vi "torres hanoi labview.vi"() -> ()   [LabVIEW 2020]
uses:
  <vilib>/Utility/miscctls.llb/LVPoint32TypeDef.ctl
  <vilib>/Utility/miscctls.llb/LVPositionTypeDef.ctl
  <vilib>/Utility/miscctls.llb/LVBoundsTypeDef.ctl
panel:
  out "Solucion del juego de 5 discos":string
  out "Boolean 3":bool
  out "Solucion del juego de 4 discos":string
  out "Boolean 2":bool
  out "Boolean":bool
  out "solucion del juego 3 discos":string
  out "Position 1":T1
  out "Position 2":T1
  out "Position 3":T1
  out "Position 4":T1
  out "Position 5":T1
  out "Position":T1
  in  "seleccione  numero de discos":u16(ring) items=["3"=3, "4"=4, "5"=5]
  out "Coords":T2
  in  "?":bool
  out "disco5":bool
  out "disco4":bool
  out "disco3":bool
  out "disco2":bool
  out "disco1":bool
  out "Torre 3":bool
  out "Torre 2":bool
  out "Torre 1":bool
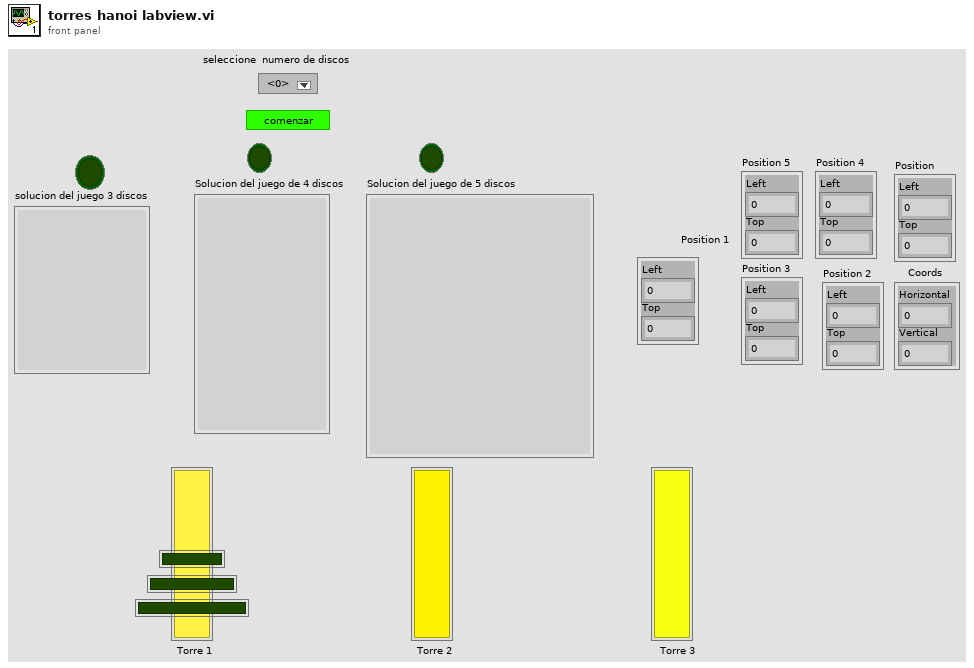
[diagram p1: front panel]
types:
  T1 = typedef "LVPositionTypeDef.ctl" = cluster{"Left":i32, "Top":i32}
  T2 = typedef "LVPoint32TypeDef.ctl" = cluster{"Horizontal":i32, "Vertical":i32}
  T3 = typedef "LVBoundsTypeDef.ctl" = cluster{"Width":u32, "Height":u32}
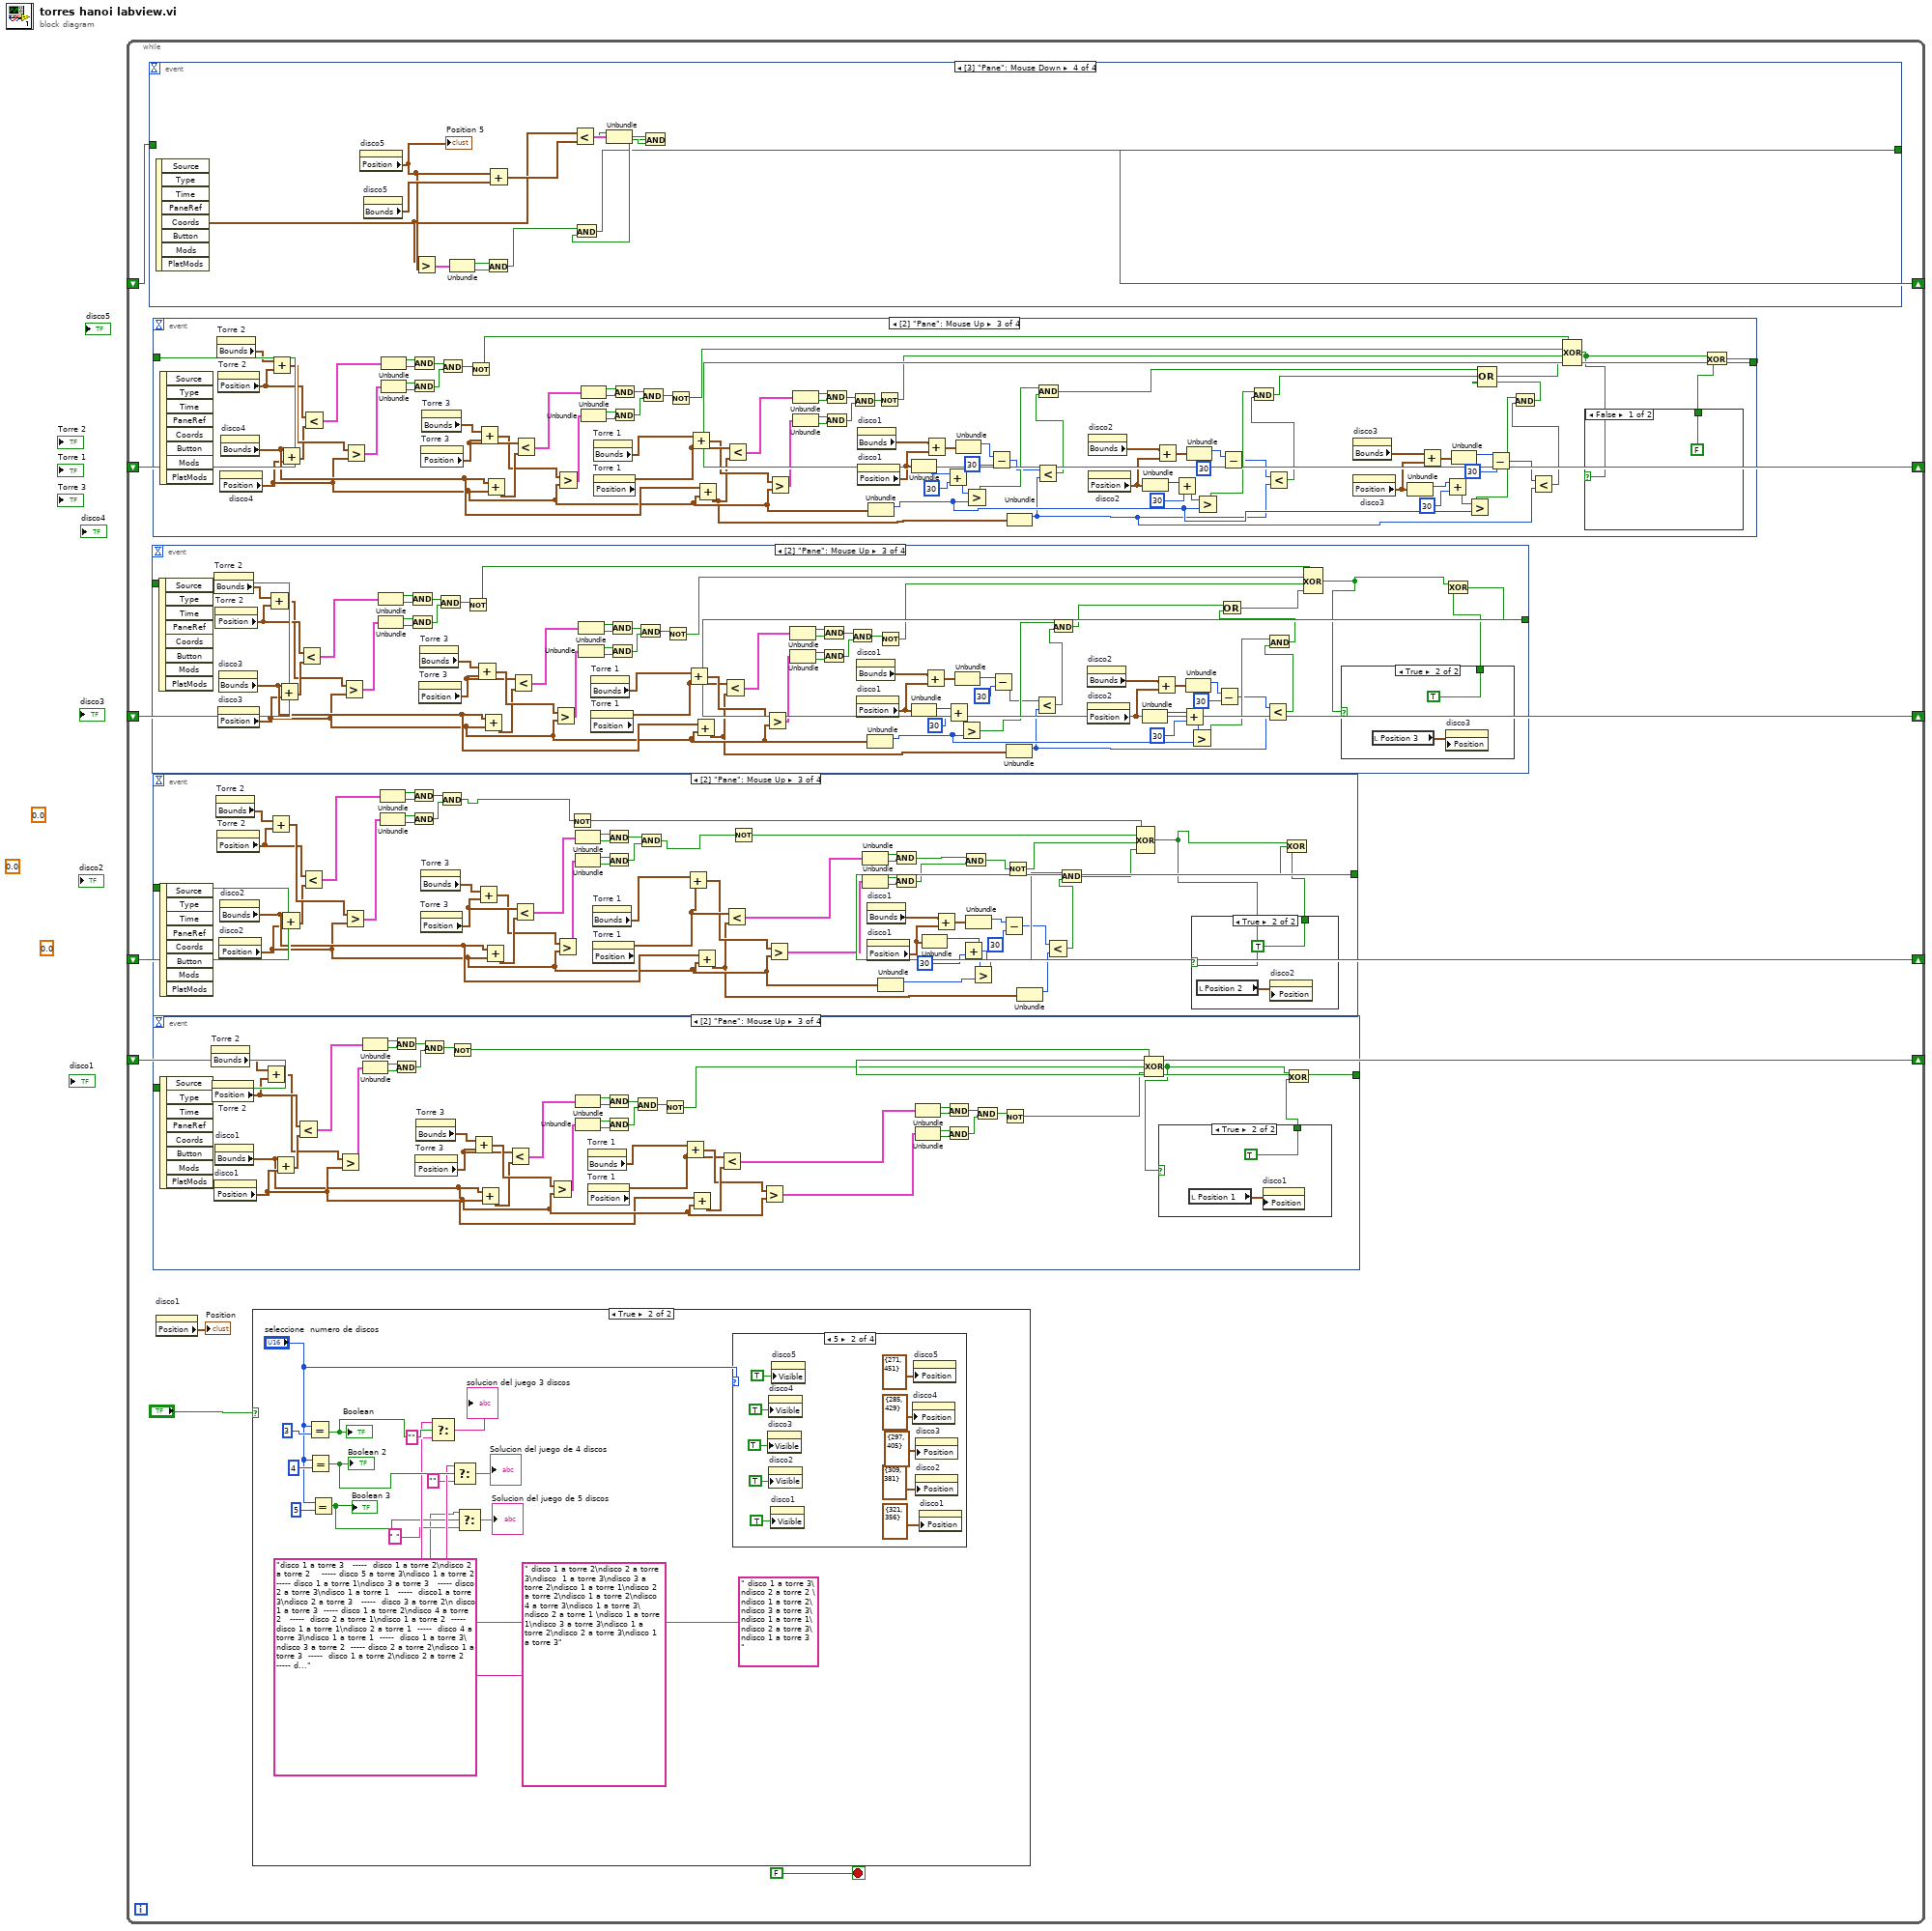
[diagram p0: block diagram]
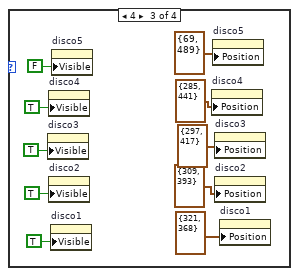
[diagram p4: hidden frame]
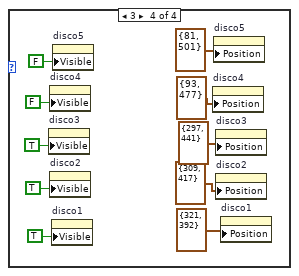
[diagram p5: hidden frame]
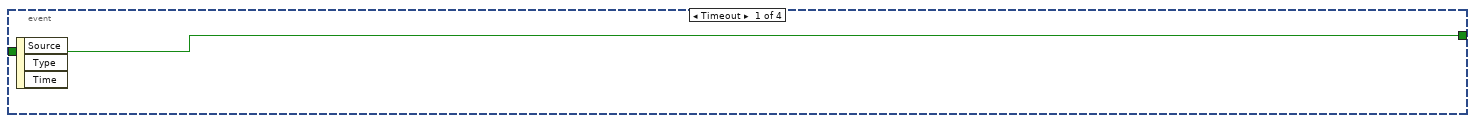
[diagram p6: hidden frame]
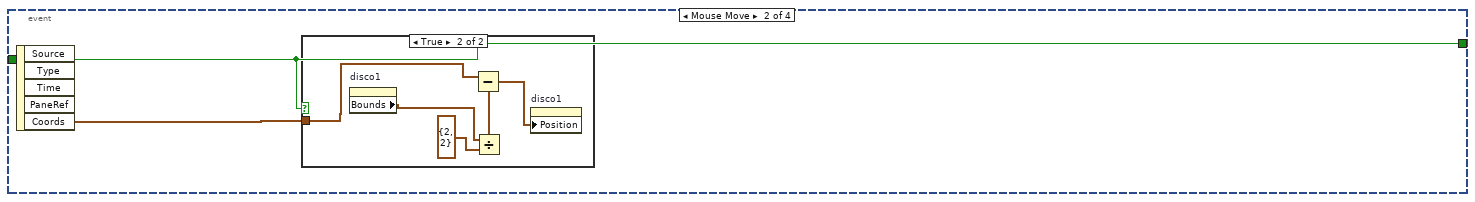
[diagram p7: hidden frame]
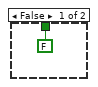
[diagram p9: hidden frame]
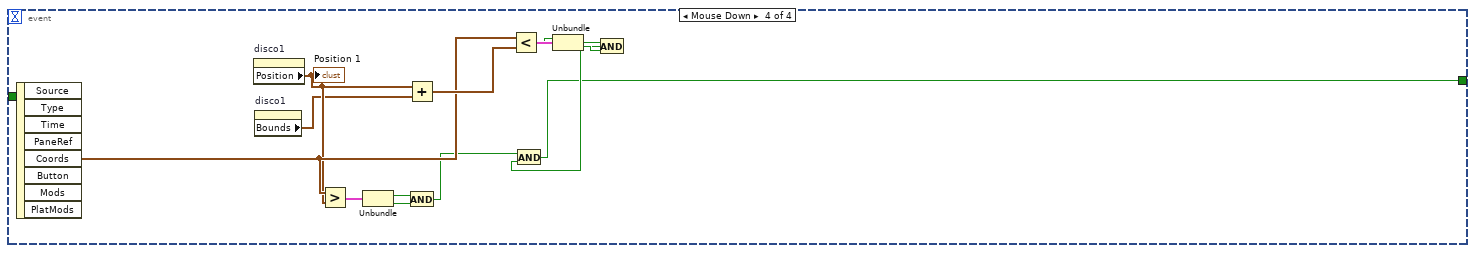
[diagram p10: hidden frame]
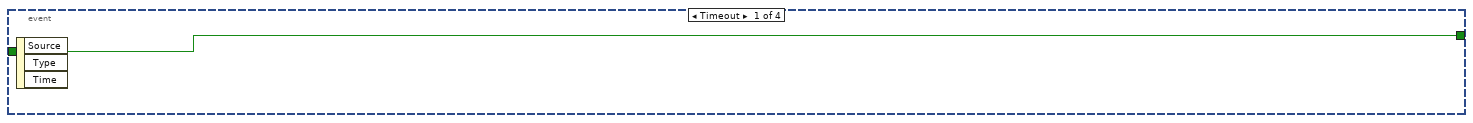
[diagram p11: hidden frame]
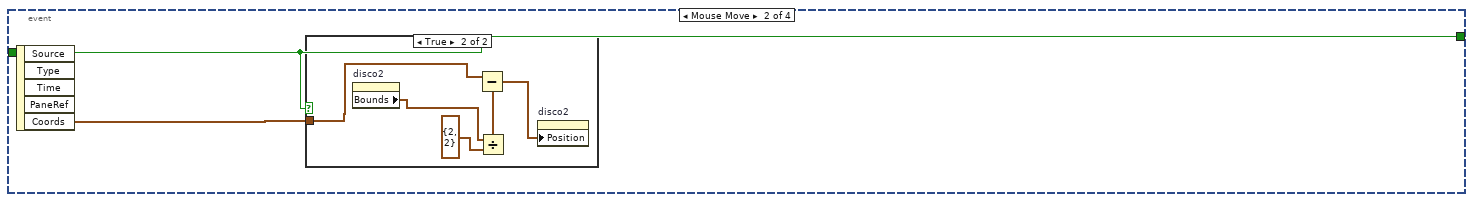
[diagram p12: hidden frame]
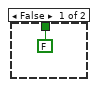
[diagram p14: hidden frame]
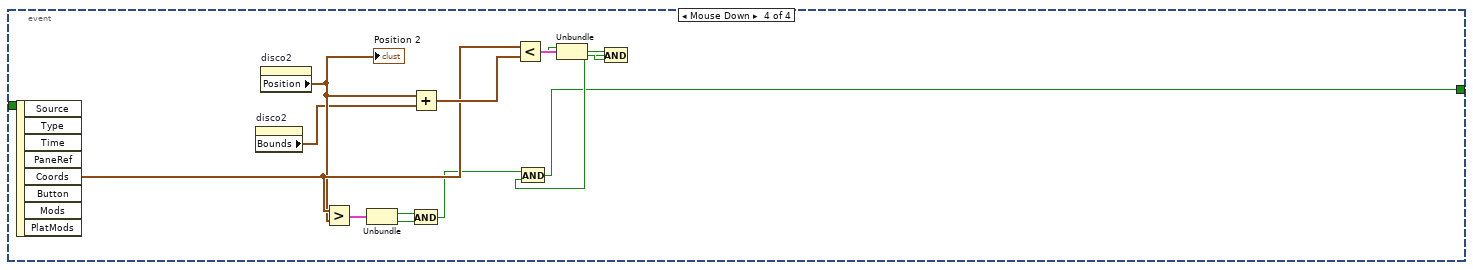
[diagram p15: hidden frame]
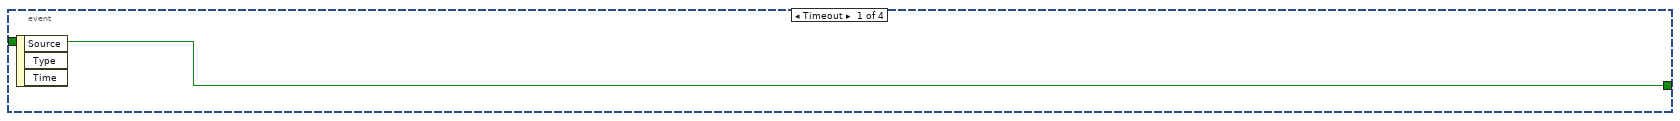
[diagram p16: hidden frame]
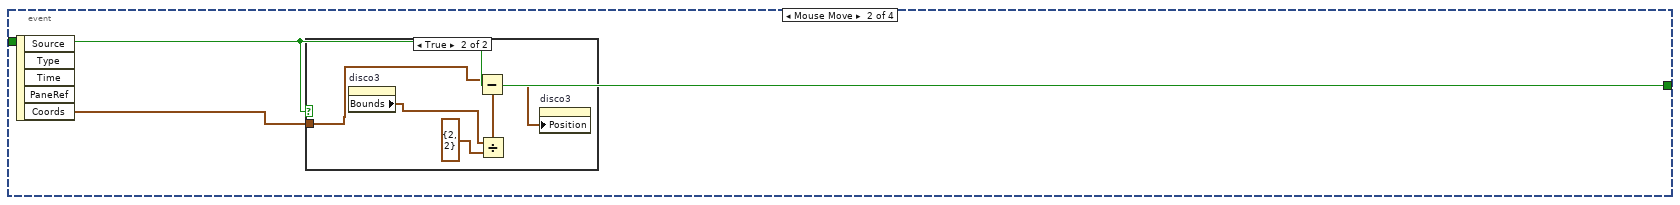
[diagram p17: hidden frame]
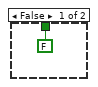
[diagram p19: hidden frame]
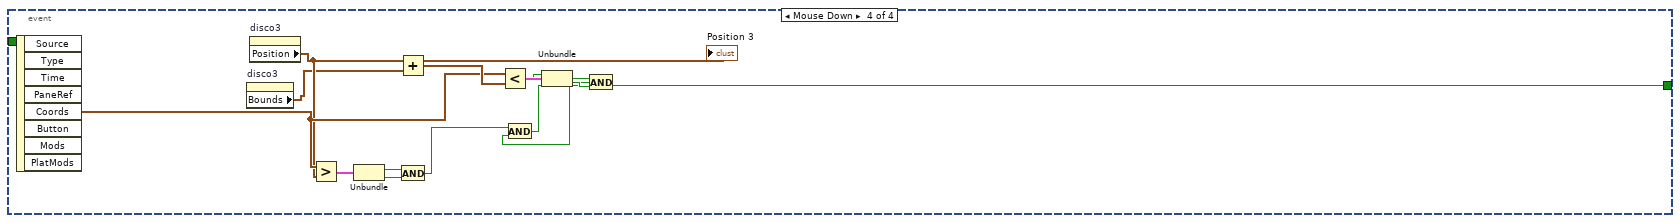
[diagram p20: hidden frame]
diagram:
  (unwired) 0.0 ("final b")
  (unwired) 0.0 ("inicio b")
  (unwired) 0.0 ("medio b")
  n1 = while {
    shift-right: [w11] -> _
    shift-left: _ -> [w12]
    shift-right: [w9] -> _
    shift-left: _ -> [w10]
    shift-right: [w7] -> _
    shift-left: _ -> [w8]
    shift-right: [w5] -> _
    shift-left: _ -> [w6]
    shift-right: [w3] -> _
    shift-left: _ -> [w4]
    stop <- FALSE stop-if-true
    n2 = event shown="[3] \"Pane\": Mouse Down" {
      selector: _ -> [_ _ _ _]
      dyn-events: _ -> [_ _ _ _]
      timeout: _ -> [_ _ _ _]
      tunnel: w12 -> [w424 w425 _ _]
      tunnel: [w424 w425 w485 w533] -> w11
      event Timeout {
        n3 = event-data() -> ()  [unwired: 1 in, 3 out]
      }
      event Mouse Move {
        n4 = event-data() -> ("Coords"=w426:T2)  [unwired: 1 in, 4 out]
        n5 = case shown="True" w425 {
          tunnel: w426 -> [_ w429]
          frame False {
          }
          frame True {
            n6 = property on="disco5" class="Bool (strict)"() -> ("Bounds"=w431:T3)  [unwired: 2 in, 2 out]
            n7 = Divide(x=w431, y=T3 {"Width"=2, "Height"=2}) -> (x/y=w428:cluster{"Width":dbl, "Height":dbl})
            n8 = Subtract(x=w429, y=w428) -> (x-y=w427:cluster{dbl, dbl})
            n9 = property on="disco5" class="Bool (strict)"("Position"=w427) -> ()  [unwired: 2 in, 2 out]
            "Coords" <- w429
          }
        }
      }
      event Mouse Up {
        n10 = event-data() -> ()  [unwired: 1 in, 8 out]
        n11 = property on="Torre 2" class="Bool (strict)"() -> ("Bounds"=w520:T3)  [unwired: 2 in, 2 out]
        n12 = property on="Torre 2" class="Bool (strict)"() -> ("Position"=w519:T1)  [unwired: 2 in, 2 out]
        n13 = property on="disco5" class="Bool (strict)"() -> ("Position"=w473:T1)  [unwired: 2 in, 2 out]
        n14 = property on="disco5" class="Bool (strict)"() -> ("Bounds"=w491:T3)  [unwired: 2 in, 2 out]
        n15 = Add(x=w520, y=w519) -> (x+y=w518:T3)
        n16 = Add(x=w491, y=w473) -> (x+y=w523:T3)
        n17 = Less?(x=w519, y=w523) -> (x < y?=w522:cluster{bool, bool})
        n18 = Greater?(x=w518, y=w473) -> (0:w521:cluster{bool, bool})
        n19 = Unbundle(w522) -> (w527:bool, w526:bool)
        n20 = Unbundle(w521) -> (w529:bool, w528:bool)
        n21 = And(x=w527, y=w526) -> (x .and. y?=w524:bool)
        n22 = And(x=w529, y=w528) -> (x .and. y?=w525:bool)
        n23 = property on="Torre 3" class="Bool (strict)"() -> ("Position"=w504:T1)  [unwired: 2 in, 2 out]
        n24 = property on="Torre 3" class="Bool (strict)"() -> ("Bounds"=w505:T3)  [unwired: 2 in, 2 out]
        n25 = And(x=w524, y=w525) -> (x .and. y?=w517:bool)
        n26 = Not(x=w517) -> (.not. x?=w488:bool)
        n27 = Add(x=w505, y=w504) -> (x+y=w515:T3)
        n28 = Add(x=w491, y=w473) -> (x+y=w512:T3)
        n29 = Less?(x=w504, y=w512) -> (x < y?=w513:cluster{bool, bool})
        n30 = Greater?(x=w515, y=w473) -> (0:w514:cluster{bool, bool})
        n31 = Unbundle(w513) -> (w508:bool, w509:bool)
        n32 = Unbundle(w514) -> (w506:bool, w507:bool)
        n33 = property on="Torre 1" class="Bool (strict)"() -> ("Bounds"=w493:T3)  [unwired: 2 in, 2 out]
        n34 = property on="Torre 1" class="Bool (strict)"() -> ("Position"=w492:T1)  [unwired: 2 in, 2 out]
        n35 = And(x=w508, y=w509) -> (x .and. y?=w511:bool)
        n36 = And(x=w506, y=w507) -> (x .and. y?=w510:bool)
        n37 = And(x=w511, y=w510) -> (x .and. y?=w516:bool)
        n38 = Not(x=w516) -> (.not. x?=w489:bool)
        n39 = Add(x=w493, y=w492) -> (x+y=w495:T3)
        n40 = Add(x=w491, y=w473) -> (x+y=w472:T3)
        n41 = Less?(x=w492, y=w472) -> (x < y?=w497:cluster{bool, bool})
        n42 = Greater?(x=w495, y=w473) -> (0:w496:cluster{bool, bool})
        n43 = Unbundle(w497) -> (w501:bool, w500:bool)
        n44 = Unbundle(w496) -> (w503:bool, w502:bool)
        n45 = property on="disco1" class="Bool (strict)"() -> ("Bounds"=w479:T3)  [unwired: 2 in, 2 out]
        n46 = property on="disco1" class="Bool (strict)"() -> ("Position"=w480:T1)  [unwired: 2 in, 2 out]
        n47 = Unbundle(w473) -> ("Left"=w462:i32)  [unwired: 1 out]
        n48 = And(x=w501, y=w500) -> (x .and. y?=w498:bool)
        n49 = And(x=w503, y=w502) -> (x .and. y?=w499:bool)
        n50 = And(x=w498, y=w499) -> (x .and. y?=w494:bool)
        n51 = Unbundle(w480) -> ("Left"=w460:i32)  [unwired: 1 out]
        n52 = Add(x=w479, y=w480) -> (x+y=w481:T3)
        n53 = Not(x=w494) -> (.not. x?=w490:bool)
        n54 = Add(x=w460, y=30) -> (x+y=w458:i32)
        n55 = Greater?(x=w458, y=w462) -> (0:w475:bool)
        n56 = Unbundle(w481) -> ("Width"=w457:u32)  [unwired: 1 out]
        n57 = Subtract(x=w457, y=u32 30) -> (x-y=w455:u32)
        n58 = Unbundle(w472) -> ("Width"=w461:u32)  [unwired: 1 out]
        n59 = Less?(x=w455, y=w461) -> (x < y?=w474:bool)
        n60 = And(x=w475, y=w474) -> (x .and. y?=w432:bool)
        n61 = property on="disco2" class="Bool (strict)"() -> ("Bounds"=w478:T3)  [unwired: 2 in, 2 out]
        n62 = property on="disco2" class="Bool (strict)"() -> ("Position"=w477:T1)  [unwired: 2 in, 2 out]
        n63 = Unbundle(w477) -> ("Left"=w453:i32)  [unwired: 1 out]
        n64 = Add(x=w478, y=w477) -> (x+y=w476:T3)
        n65 = Add(x=w453, y=30) -> (x+y=w454:i32)
        n66 = Unbundle(w476) -> ("Width"=w451:u32)  [unwired: 1 out]
        n67 = Greater?(x=w454, y=w462) -> (0:w471:bool)
        n68 = Subtract(x=w451, y=u32 30) -> (x-y=w450:u32)
        n69 = Less?(x=w450, y=w461) -> (x < y?=w470:bool)
        n70 = And(x=w471, y=w470) -> (x .and. y?=w433:bool)
        n71 = property on="disco3" class="Bool (strict)"() -> ("Bounds"=w482:T3)  [unwired: 2 in, 2 out]
        n72 = property on="disco3" class="Bool (strict)"() -> ("Position"=w483:T1)  [unwired: 2 in, 2 out]
        n73 = Unbundle(w483) -> ("Left"=w448:i32)  [unwired: 1 out]
        n74 = Add(x=w482, y=w483) -> (x+y=w484:T3)
        n75 = Add(x=w448, y=30) -> (x+y=w447:i32)
        n76 = Unbundle(w484) -> ("Width"=w445:u32)  [unwired: 1 out]
        n77 = Greater?(x=w447, y=w462) -> (0:w469:bool)
        n78 = Subtract(x=w445, y=u32 30) -> (x-y=w444:u32)
        n79 = Less?(x=w444, y=w461) -> (x < y?=w468:bool)
        n80 = And(x=w469, y=w468) -> (x .and. y?=w434:bool)
        n81 = property on="disco4" class="Bool (strict)"() -> ("Bounds"=w465:T3)  [unwired: 2 in, 2 out]
        n82 = property on="disco4" class="Bool (strict)"() -> ("Position"=w464:T1)  [unwired: 2 in, 2 out]
        n83 = Unbundle(w464) -> ("Left"=w442:i32)  [unwired: 1 out]
        n84 = Add(x=w465, y=w464) -> (x+y=w463:T3)
        n85 = Add(x=w442, y=30) -> (x+y=w441:i32)
        n86 = Greater?(x=w441, y=w462) -> (0:w466:bool)
        n87 = Unbundle(w463) -> ("Width"=w439:u32)  [unwired: 1 out]
        n88 = Subtract(x=w439, y=u32 30) -> (x-y=w437:u32)
        n89 = Less?(x=w437, y=w461) -> (x < y?=w467:bool)
        n90 = And(x=w466, y=w467) -> (x .and. y?=w435:bool)
        n91 = Compound Arithmetic op=OR(w432, w433, w434, w435) -> (w436:bool)
        n92 = Compound Arithmetic op=XOR(w488, w489, w490, w436) -> (w486:bool)
        n93 = case shown="True" w486 {
          tunnel: [FALSE ("Accepted?") TRUE ("Accepted?")] -> w487
          frame False {
          }
          frame True {
            n94 = local read "Position 5"() -> (w532:T1)
            n95 = property on="disco5" class="Bool (strict)"("Position"=w532) -> ()  [unwired: 2 in, 2 out]
          }
        }
        n96 = Exclusive Or(1:w487, 2:w486) -> (0:w485:bool)
      }
      event Mouse Down {
        n97 = event-data() -> ("Coords"=w542:T2)  [unwired: 1 in, 7 out]
        n98 = property on="disco5" class="Bool (strict)"() -> ("Position"=w544:T1)  [unwired: 2 in, 2 out]
        "Position 5" <- w544
        n99 = property on="disco5" class="Bool (strict)"() -> ("Bounds"=w545:T3)  [unwired: 2 in, 2 out]
        n100 = Greater?(x=w542, y=w544) -> (0:w541:cluster{bool, bool})
        n101 = Unbundle(w541) -> (w537:bool, w536:bool)
        n102 = Add(x=w544, y=w545) -> (x+y=w543:T3)
        n103 = And(x=w537, y=w536) -> (x .and. y?=w534:bool)
        n104 = Less?(x=w542, y=w543) -> (x < y?=w540:cluster{bool, bool})
        n105 = Unbundle(w540) -> (w539:bool, w538:bool)
        n106 = And(x=w539, y=w538) -> (x .and. y?=w535:bool)
        n107 = And(x=w534, y=w535) -> (x .and. y?=w533:bool)
      }
    }
    n108 = event shown="[2] \"Pane\": Mouse Up" {
      selector: _ -> [_ _ _ _]
      dyn-events: _ -> [_ _ _ _]
      timeout: _ -> [_ _ _ _]
      tunnel: w8 -> [w216 w217 _ _]
      tunnel: [w216 w217 w253 w303] -> w7
      event Timeout {
        n109 = event-data() -> ()  [unwired: 1 in, 3 out]
      }
      event Mouse Move {
        n110 = event-data() -> ("Coords"=w218:T2)  [unwired: 1 in, 4 out]
        n111 = case shown="True" w217 {
          tunnel: w218 -> [_ w222]
          frame False {
          }
          frame True {
            n112 = property on="disco3" class="Bool (strict)"() -> ("Bounds"=w220:T3)  [unwired: 2 in, 2 out]
            n113 = Divide(x=w220, y=T3 {"Width"=2, "Height"=2}) -> (x/y=w221:cluster{"Width":dbl, "Height":dbl})
            n114 = Subtract(x=w222, y=w221) -> (x-y=w219:cluster{dbl, dbl})
            n115 = property on="disco3" class="Bool (strict)"("Position"=w219) -> ()  [unwired: 2 in, 2 out]
          }
        }
      }
      event Mouse Up {
        n116 = event-data() -> ()  [unwired: 1 in, 8 out]
        n117 = property on="Torre 2" class="Bool (strict)"() -> ("Bounds"=w288:T3)  [unwired: 2 in, 2 out]
        n118 = property on="Torre 2" class="Bool (strict)"() -> ("Position"=w287:T1)  [unwired: 2 in, 2 out]
        n119 = property on="disco3" class="Bool (strict)"() -> ("Position"=w249:T1)  [unwired: 2 in, 2 out]
        n120 = property on="disco3" class="Bool (strict)"() -> ("Bounds"=w259:T3)  [unwired: 2 in, 2 out]
        n121 = Add(x=w288, y=w287) -> (x+y=w286:T3)
        n122 = Add(x=w259, y=w249) -> (x+y=w291:T3)
        n123 = Less?(x=w287, y=w291) -> (x < y?=w290:cluster{bool, bool})
        n124 = Greater?(x=w286, y=w249) -> (0:w289:cluster{bool, bool})
        n125 = Unbundle(w290) -> (w295:bool, w294:bool)
        n126 = Unbundle(w289) -> (w297:bool, w296:bool)
        n127 = And(x=w295, y=w294) -> (x .and. y?=w292:bool)
        n128 = And(x=w297, y=w296) -> (x .and. y?=w293:bool)
        n129 = property on="Torre 3" class="Bool (strict)"() -> ("Position"=w272:T1)  [unwired: 2 in, 2 out]
        n130 = property on="Torre 3" class="Bool (strict)"() -> ("Bounds"=w273:T3)  [unwired: 2 in, 2 out]
        n131 = And(x=w292, y=w293) -> (x .and. y?=w285:bool)
        n132 = Not(x=w285) -> (.not. x?=w256:bool)
        n133 = Add(x=w273, y=w272) -> (x+y=w283:T3)
        n134 = Add(x=w259, y=w249) -> (x+y=w280:T3)
        n135 = Less?(x=w272, y=w280) -> (x < y?=w281:cluster{bool, bool})
        n136 = Greater?(x=w283, y=w249) -> (0:w282:cluster{bool, bool})
        n137 = Unbundle(w281) -> (w276:bool, w277:bool)
        n138 = Unbundle(w282) -> (w274:bool, w275:bool)
        n139 = property on="Torre 1" class="Bool (strict)"() -> ("Bounds"=w261:T3)  [unwired: 2 in, 2 out]
        n140 = property on="Torre 1" class="Bool (strict)"() -> ("Position"=w260:T1)  [unwired: 2 in, 2 out]
        n141 = And(x=w276, y=w277) -> (x .and. y?=w279:bool)
        n142 = And(x=w274, y=w275) -> (x .and. y?=w278:bool)
        n143 = And(x=w279, y=w278) -> (x .and. y?=w284:bool)
        n144 = Not(x=w284) -> (.not. x?=w257:bool)
        n145 = Add(x=w261, y=w260) -> (x+y=w263:T3)
        n146 = Add(x=w259, y=w249) -> (x+y=w248:T3)
        n147 = Less?(x=w260, y=w248) -> (x < y?=w265:cluster{bool, bool})
        n148 = Greater?(x=w263, y=w249) -> (0:w264:cluster{bool, bool})
        n149 = Unbundle(w265) -> (w269:bool, w268:bool)
        n150 = Unbundle(w264) -> (w271:bool, w270:bool)
        n151 = And(x=w269, y=w268) -> (x .and. y?=w266:bool)
        n152 = And(x=w271, y=w270) -> (x .and. y?=w267:bool)
        n153 = And(x=w266, y=w267) -> (x .and. y?=w262:bool)
        n154 = property on="disco1" class="Bool (strict)"() -> ("Bounds"=w250:T3)  [unwired: 2 in, 2 out]
        n155 = property on="disco1" class="Bool (strict)"() -> ("Position"=w251:T1)  [unwired: 2 in, 2 out]
        n156 = Unbundle(w249) -> ("Left"=w242:i32)  [unwired: 1 out]
        n157 = Not(x=w262) -> (.not. x?=w258:bool)
        n158 = Unbundle(w251) -> ("Left"=w238:i32)  [unwired: 1 out]
        n159 = Add(x=w250, y=w251) -> (x+y=w252:T3)
        n160 = Add(x=w238, y=30) -> (x+y=w237:i32)
        n161 = Unbundle(w252) -> ("Width"=w234:u32)  [unwired: 1 out]
        n162 = Greater?(x=w237, y=w242) -> (0:w247:bool)
        n163 = Subtract(x=w234, y=u32 30) -> (x-y=w235:u32)
        n164 = Unbundle(w248) -> ("Width"=w241:u32)  [unwired: 1 out]
        n165 = Less?(x=w235, y=w241) -> (x < y?=w246:bool)
        n166 = And(x=w247, y=w246) -> (x .and. y?=w225:bool)
        n167 = property on="disco2" class="Bool (strict)"() -> ("Bounds"=w245:T3)  [unwired: 2 in, 2 out]
        n168 = property on="disco2" class="Bool (strict)"() -> ("Position"=w244:T1)  [unwired: 2 in, 2 out]
        n169 = Unbundle(w244) -> ("Left"=w232:i32)  [unwired: 1 out]
        n170 = Add(x=w245, y=w244) -> (x+y=w243:T3)
        n171 = Add(x=w232, y=30) -> (x+y=w231:i32)
        n172 = Unbundle(w243) -> ("Width"=w229:u32)  [unwired: 1 out]
        n173 = Greater?(x=w231, y=w242) -> (0:w239:bool)
        n174 = Subtract(x=w229, y=u32 30) -> (x-y=w228:u32)
        n175 = Less?(x=w228, y=w241) -> (x < y?=w240:bool)
        n176 = And(x=w239, y=w240) -> (x .and. y?=w226:bool)
        n177 = Or(x=w225, y=w226) -> (x .or. y?=w224:bool)
        n178 = Compound Arithmetic op=XOR(w256, w257, w258, w224) -> (w254:bool)
        n179 = case shown="True" w254 {
          tunnel: [FALSE ("Accepted?") TRUE ("Accepted?")] -> w255
          frame False {
          }
          frame True {
            n180 = local read "Position 3"() -> (w300:T1)
            n181 = property on="disco3" class="Bool (strict)"("Position"=w300) -> ()  [unwired: 2 in, 2 out]
          }
        }
        n182 = Exclusive Or(1:w255, 2:w254) -> (0:w253:bool)
      }
      event Mouse Down {
        n183 = event-data() -> ("Coords"=w312:T2)  [unwired: 1 in, 7 out]
        n184 = property on="disco3" class="Bool (strict)"() -> ("Bounds"=w301:T3)  [unwired: 2 in, 2 out]
        n185 = property on="disco3" class="Bool (strict)"() -> ("Position"=w302:T1)  [unwired: 2 in, 2 out]
        "Position 3" <- w302
        n186 = Greater?(x=w312, y=w302) -> (0:w311:cluster{bool, bool})
        n187 = Unbundle(w311) -> (w307:bool, w306:bool)
        n188 = Add(x=w302, y=w301) -> (x+y=w313:T3)
        n189 = And(x=w307, y=w306) -> (x .and. y?=w304:bool)
        n190 = Less?(x=w312, y=w313) -> (x < y?=w310:cluster{bool, bool})
        n191 = Unbundle(w310) -> (w309:bool, w308:bool)
        n192 = And(x=w309, y=w308) -> (x .and. y?=w305:bool)
        n193 = And(x=w304, y=w305) -> (x .and. y?=w303:bool)
      }
    }
    n194 = event shown="[2] \"Pane\": Mouse Up" {
      selector: _ -> [_ _ _ _]
      dyn-events: _ -> [_ _ _ _]
      timeout: _ -> [_ _ _ _]
      tunnel: w10 -> [w314 w315 _ _]
      tunnel: [w314 w315 w364 w413] -> w9
      event Timeout {
        n195 = event-data() -> ()  [unwired: 1 in, 3 out]
      }
      event Mouse Move {
        n196 = event-data() -> ("Coords"=w316:T2)  [unwired: 1 in, 4 out]
        n197 = case shown="True" w315 {
          tunnel: w316 -> [_ w317]
          frame False {
          }
          frame True {
            n198 = property on="disco4" class="Bool (strict)"() -> ("Bounds"=w319:T3)  [unwired: 2 in, 2 out]
            n199 = Divide(x=w319, y=T3 {"Width"=2, "Height"=2}) -> (x/y=w320:cluster{"Width":dbl, "Height":dbl})
            n200 = Subtract(x=w317, y=w320) -> (x-y=w318:cluster{dbl, dbl})
            n201 = property on="disco4" class="Bool (strict)"("Position"=w318) -> ()  [unwired: 2 in, 2 out]
          }
        }
      }
      event Mouse Up {
        n202 = event-data() -> ()  [unwired: 1 in, 8 out]
        n203 = property on="Torre 2" class="Bool (strict)"() -> ("Bounds"=w374:T3)  [unwired: 2 in, 2 out]
        n204 = property on="Torre 2" class="Bool (strict)"() -> ("Position"=w375:T1)  [unwired: 2 in, 2 out]
        n205 = property on="disco4" class="Bool (strict)"() -> ("Position"=w353:T1)  [unwired: 2 in, 2 out]
        n206 = property on="disco4" class="Bool (strict)"() -> ("Bounds"=w403:T3)  [unwired: 2 in, 2 out]
        n207 = Add(x=w374, y=w375) -> (x+y=w376:T3)
        n208 = Add(x=w403, y=w353) -> (x+y=w371:T3)
        n209 = Less?(x=w375, y=w371) -> (x < y?=w372:cluster{bool, bool})
        n210 = Greater?(x=w376, y=w353) -> (0:w373:cluster{bool, bool})
        n211 = Unbundle(w372) -> (w367:bool, w368:bool)
        n212 = Unbundle(w373) -> (w365:bool, w366:bool)
        n213 = And(x=w367, y=w368) -> (x .and. y?=w370:bool)
        n214 = And(x=w365, y=w366) -> (x .and. y?=w369:bool)
        n215 = property on="Torre 3" class="Bool (strict)"() -> ("Position"=w390:T1)  [unwired: 2 in, 2 out]
        n216 = property on="Torre 3" class="Bool (strict)"() -> ("Bounds"=w389:T3)  [unwired: 2 in, 2 out]
        n217 = And(x=w370, y=w369) -> (x .and. y?=w377:bool)
        n218 = Not(x=w377) -> (.not. x?=w405:bool)
        n219 = Add(x=w389, y=w390) -> (x+y=w379:T3)
        n220 = Add(x=w403, y=w353) -> (x+y=w382:T3)
        n221 = Less?(x=w390, y=w382) -> (x < y?=w381:cluster{bool, bool})
        n222 = Greater?(x=w379, y=w353) -> (0:w380:cluster{bool, bool})
        n223 = Unbundle(w381) -> (w386:bool, w385:bool)
        n224 = Unbundle(w380) -> (w388:bool, w387:bool)
        n225 = property on="Torre 1" class="Bool (strict)"() -> ("Bounds"=w401:T3)  [unwired: 2 in, 2 out]
        n226 = property on="Torre 1" class="Bool (strict)"() -> ("Position"=w402:T1)  [unwired: 2 in, 2 out]
        n227 = And(x=w386, y=w385) -> (x .and. y?=w383:bool)
        n228 = And(x=w388, y=w387) -> (x .and. y?=w384:bool)
        n229 = And(x=w383, y=w384) -> (x .and. y?=w378:bool)
        n230 = Not(x=w378) -> (.not. x?=w404:bool)
        n231 = Add(x=w401, y=w402) -> (x+y=w399:T3)
        n232 = Add(x=w403, y=w353) -> (x+y=w352:T3)
        n233 = Less?(x=w402, y=w352) -> (x < y?=w397:cluster{bool, bool})
        n234 = Greater?(x=w399, y=w353) -> (0:w398:cluster{bool, bool})
        n235 = Unbundle(w397) -> (w393:bool, w394:bool)
        n236 = Unbundle(w398) -> (w391:bool, w392:bool)
        n237 = And(x=w393, y=w394) -> (x .and. y?=w396:bool)
        n238 = And(x=w391, y=w392) -> (x .and. y?=w395:bool)
        n239 = And(x=w396, y=w395) -> (x .and. y?=w400:bool)
        n240 = property on="disco1" class="Bool (strict)"() -> ("Bounds"=w360:T3)  [unwired: 2 in, 2 out]
        n241 = property on="disco1" class="Bool (strict)"() -> ("Position"=w359:T1)  [unwired: 2 in, 2 out]
        n242 = Unbundle(w353) -> ("Left"=w348:i32)  [unwired: 1 out]
        n243 = Not(x=w400) -> (.not. x?=w323:bool)
        n244 = Unbundle(w359) -> ("Left"=w344:i32)  [unwired: 1 out]
        n245 = Add(x=w360, y=w359) -> (x+y=w358:T3)
        n246 = Add(x=w344, y=30) -> (x+y=w342:i32)
        n247 = Unbundle(w358) -> ("Width"=w341:u32)  [unwired: 1 out]
        n248 = Greater?(x=w342, y=w348) -> (0:w355:bool)
        n249 = Subtract(x=w341, y=u32 30) -> (x-y=w340:u32)
        n250 = Unbundle(w352) -> ("Width"=w347:u32)  [unwired: 1 out]
        n251 = Less?(x=w340, y=w347) -> (x < y?=w354:bool)
        n252 = And(x=w355, y=w354) -> (x .and. y?=w324:bool)
        n253 = property on="disco2" class="Bool (strict)"() -> ("Bounds"=w361:T3)  [unwired: 2 in, 2 out]
        n254 = property on="disco2" class="Bool (strict)"() -> ("Position"=w362:T1)  [unwired: 2 in, 2 out]
        n255 = Unbundle(w362) -> ("Left"=w337:i32)  [unwired: 1 out]
        n256 = Add(x=w361, y=w362) -> (x+y=w363:T3)
        n257 = Add(x=w337, y=30) -> (x+y=w338:i32)
        n258 = Unbundle(w363) -> ("Width"=w335:u32)  [unwired: 1 out]
        n259 = Greater?(x=w338, y=w348) -> (0:w357:bool)
        n260 = Subtract(x=w335, y=u32 30) -> (x-y=w333:u32)
        n261 = Less?(x=w333, y=w347) -> (x < y?=w356:bool)
        n262 = And(x=w357, y=w356) -> (x .and. y?=w325:bool)
        n263 = property on="disco3" class="Bool (strict)"() -> ("Bounds"=w351:T3)  [unwired: 2 in, 2 out]
        n264 = property on="disco3" class="Bool (strict)"() -> ("Position"=w350:T1)  [unwired: 2 in, 2 out]
        n265 = Unbundle(w350) -> ("Left"=w332:i32)  [unwired: 1 out]
        n266 = Add(x=w351, y=w350) -> (x+y=w349:T3)
        n267 = Add(x=w332, y=30) -> (x+y=w331:i32)
        n268 = Unbundle(w349) -> ("Width"=w329:u32)  [unwired: 1 out]
        n269 = Greater?(x=w331, y=w348) -> (0:w346:bool)
        n270 = Subtract(x=w329, y=u32 30) -> (x-y=w328:u32)
        n271 = Less?(x=w328, y=w347) -> (x < y?=w345:bool)
        n272 = And(x=w346, y=w345) -> (x .and. y?=w326:bool)
        n273 = Compound Arithmetic op=OR(w324, w325, w326) -> (w322:bool)
        n274 = Compound Arithmetic op=XOR(w405, w404, w323, w322) -> (w407:bool)
        n275 = case shown="False" w407 {
          tunnel: [FALSE ("Accepted?") TRUE ("Accepted?")] -> w406
          frame False {
          }
          frame True {
            n276 = local read "Position 4"() -> (w410:T1)
            n277 = property on="disco4" class="Bool (strict)"("Position"=w410) -> ()  [unwired: 2 in, 2 out]
          }
        }
        n278 = Exclusive Or(1:w406, 2:w407) -> (0:w364:bool)
      }
      event Mouse Down {
        n279 = event-data() -> ("Coords"=w422:T2)  [unwired: 1 in, 7 out]
        n280 = property on="disco4" class="Bool (strict)"() -> ("Position"=w412:T1)  [unwired: 2 in, 2 out]
        "Position 4" <- w412
        n281 = property on="disco4" class="Bool (strict)"() -> ("Bounds"=w411:T3)  [unwired: 2 in, 2 out]
        n282 = Greater?(x=w422, y=w412) -> (0:w421:cluster{bool, bool})
        n283 = Unbundle(w421) -> (w417:bool, w416:bool)
        n284 = Add(x=w412, y=w411) -> (x+y=w423:T3)
        n285 = And(x=w417, y=w416) -> (x .and. y?=w414:bool)
        n286 = Less?(x=w422, y=w423) -> (x < y?=w420:cluster{bool, bool})
        n287 = Unbundle(w420) -> (w419:bool, w418:bool)
        n288 = And(x=w419, y=w418) -> (x .and. y?=w415:bool)
        n289 = And(x=w414, y=w415) -> (x .and. y?=w413:bool)
      }
    }
    n290 = event shown="[2] \"Pane\": Mouse Up" {
      selector: _ -> [_ _ _ _]
      dyn-events: _ -> [_ _ _ _]
      timeout: _ -> [_ _ _ _]
      tunnel: w6 -> [w131 w132 _ _]
      tunnel: [w131 w132 w159 w205] -> w5
      event Timeout {
        n291 = event-data() -> ()  [unwired: 1 in, 3 out]
      }
      event Mouse Move {
        n292 = event-data() -> ("Coords"=w133:T2)  [unwired: 1 in, 4 out]
        n293 = case shown="True" w132 {
          tunnel: w133 -> [_ w137]
          frame False {
          }
          frame True {
            n294 = property on="disco2" class="Bool (strict)"() -> ("Bounds"=w135:T3)  [unwired: 2 in, 2 out]
            n295 = Divide(x=w135, y=T3 {"Width"=2, "Height"=2}) -> (x/y=w136:cluster{"Width":dbl, "Height":dbl})
            n296 = Subtract(x=w137, y=w136) -> (x-y=w134:cluster{dbl, dbl})
            n297 = property on="disco2" class="Bool (strict)"("Position"=w134) -> ()  [unwired: 2 in, 2 out]
          }
        }
      }
      event Mouse Up {
        n298 = event-data() -> ()  [unwired: 1 in, 8 out]
        n299 = property on="Torre 2" class="Bool (strict)"() -> ("Bounds"=w169:T3)  [unwired: 2 in, 2 out]
        n300 = property on="Torre 2" class="Bool (strict)"() -> ("Position"=w170:T1)  [unwired: 2 in, 2 out]
        n301 = property on="disco2" class="Bool (strict)"() -> ("Position"=w154:T1)  [unwired: 2 in, 2 out]
        n302 = property on="disco2" class="Bool (strict)"() -> ("Bounds"=w195:T3)  [unwired: 2 in, 2 out]
        n303 = Add(x=w169, y=w170) -> (x+y=w171:T3)
        n304 = Add(x=w195, y=w154) -> (x+y=w166:T3)
        n305 = Less?(x=w170, y=w166) -> (x < y?=w167:cluster{bool, bool})
        n306 = Greater?(x=w171, y=w154) -> (0:w168:cluster{bool, bool})
        n307 = Unbundle(w167) -> (w162:bool, w163:bool)
        n308 = Unbundle(w168) -> (w160:bool, w161:bool)
        n309 = And(x=w162, y=w163) -> (x .and. y?=w165:bool)
        n310 = And(x=w160, y=w161) -> (x .and. y?=w164:bool)
        n311 = property on="Torre 3" class="Bool (strict)"() -> ("Position"=w183:T1)  [unwired: 2 in, 2 out]
        n312 = property on="Torre 3" class="Bool (strict)"() -> ("Bounds"=w182:T3)  [unwired: 2 in, 2 out]
        n313 = And(x=w165, y=w164) -> (x .and. y?=w157:bool)
        n314 = Add(x=w182, y=w183) -> (x+y=w172:T3)
        n315 = Add(x=w195, y=w154) -> (x+y=w175:T3)
        n316 = Less?(x=w183, y=w175) -> (x < y?=w174:cluster{bool, bool})
        n317 = Greater?(x=w172, y=w154) -> (0:w173:cluster{bool, bool})
        n318 = Not(x=w157) -> (.not. x?=w197:bool)
        n319 = Unbundle(w174) -> (w179:bool, w178:bool)
        n320 = Unbundle(w173) -> (w181:bool, w180:bool)
        n321 = property on="Torre 1" class="Bool (strict)"() -> ("Bounds"=w193:T3)  [unwired: 2 in, 2 out]
        n322 = property on="Torre 1" class="Bool (strict)"() -> ("Position"=w194:T1)  [unwired: 2 in, 2 out]
        n323 = And(x=w179, y=w178) -> (x .and. y?=w176:bool)
        n324 = And(x=w181, y=w180) -> (x .and. y?=w177:bool)
        n325 = And(x=w176, y=w177) -> (x .and. y?=w156:bool)
        n326 = Add(x=w193, y=w194) -> (x+y=w192:T3)
        n327 = Add(x=w195, y=w154) -> (x+y=w150:T3)
        n328 = Less?(x=w194, y=w150) -> (x < y?=w190:cluster{bool, bool})
        n329 = Not(x=w156) -> (.not. x?=w158:bool)
        n330 = Greater?(x=w192, y=w154) -> (0:w191:cluster{bool, bool})
        n331 = Unbundle(w190) -> (w186:bool, w187:bool)
        n332 = Unbundle(w191) -> (w184:bool, w185:bool)
        n333 = property on="disco1" class="Bool (strict)"() -> ("Bounds"=w153:T3)  [unwired: 2 in, 2 out]
        n334 = property on="disco1" class="Bool (strict)"() -> ("Position"=w152:T1)  [unwired: 2 in, 2 out]
        n335 = Unbundle(w154) -> ("Left"=w145:i32)  [unwired: 1 out]
        n336 = And(x=w186, y=w187) -> (x .and. y?=w189:bool)
        n337 = And(x=w184, y=w185) -> (x .and. y?=w188:bool)
        n338 = Unbundle(w152) -> ("Left"=w144:i32)  [unwired: 1 out]
        n339 = Add(x=w153, y=w152) -> (x+y=w151:T3)
        n340 = Add(x=w144, y=30) -> (x+y=w142:i32)
        n341 = And(x=w189, y=w188) -> (x .and. y?=w155:bool)
        n342 = Unbundle(w151) -> ("Width"=w140:u32)  [unwired: 1 out]
        n343 = Greater?(x=w142, y=w145) -> (0:w148:bool)
        n344 = Subtract(x=w140, y=u32 30) -> (x-y=w141:u32)
        n345 = Not(x=w155) -> (.not. x?=w196:bool)
        n346 = Unbundle(w150) -> ("Width"=w149:u32)  [unwired: 1 out]
        n347 = Less?(x=w141, y=w149) -> (x < y?=w147:bool)
        n348 = And(x=w148, y=w147) -> (x .and. y?=w146:bool)
        n349 = Compound Arithmetic op=XOR(w197, w158, w196, w146) -> (w199:bool)
        n350 = case shown="True" w199 {
          tunnel: [FALSE ("Accepted?") TRUE ("Accepted?")] -> w198
          frame False {
          }
          frame True {
            n351 = local read "Position 2"() -> (w202:T1)
            n352 = property on="disco2" class="Bool (strict)"("Position"=w202) -> ()  [unwired: 2 in, 2 out]
          }
        }
        n353 = Exclusive Or(1:w198, 2:w199) -> (0:w159:bool)
      }
      event Mouse Down {
        n354 = event-data() -> ("Coords"=w214:T2)  [unwired: 1 in, 7 out]
        n355 = property on="disco2" class="Bool (strict)"() -> ("Bounds"=w203:T3)  [unwired: 2 in, 2 out]
        n356 = property on="disco2" class="Bool (strict)"() -> ("Position"=w204:T1)  [unwired: 2 in, 2 out]
        "Position 2" <- w204
        n357 = Greater?(x=w214, y=w204) -> (0:w213:cluster{bool, bool})
        n358 = Unbundle(w213) -> (w209:bool, w208:bool)
        n359 = Add(x=w204, y=w203) -> (x+y=w215:T3)
        n360 = And(x=w209, y=w208) -> (x .and. y?=w206:bool)
        n361 = Less?(x=w214, y=w215) -> (x < y?=w212:cluster{bool, bool})
        n362 = Unbundle(w212) -> (w211:bool, w210:bool)
        n363 = And(x=w211, y=w210) -> (x .and. y?=w207:bool)
        n364 = And(x=w206, y=w207) -> (x .and. y?=w205:bool)
      }
    }
    n365 = event shown="[2] \"Pane\": Mouse Up" {
      selector: _ -> [_ _ _ _]
      dyn-events: _ -> [_ _ _ _]
      timeout: _ -> [_ _ _ _]
      tunnel: w4 -> [w60 w61 _ _]
      tunnel: [w60 w61 w71 w120] -> w3
      event Timeout {
        n366 = event-data() -> ()  [unwired: 1 in, 3 out]
      }
      event Mouse Move {
        n367 = event-data() -> ("Coords"=w62:T2)  [unwired: 1 in, 4 out]
        n368 = case shown="True" w61 {
          tunnel: w62 -> [_ w66]
          frame False {
          }
          frame True {
            n369 = property on="disco1" class="Bool (strict)"() -> ("Bounds"=w64:T3)  [unwired: 2 in, 2 out]
            n370 = Divide(x=w64, y=T3 {"Width"=2, "Height"=2}) -> (x/y=w65:cluster{"Width":dbl, "Height":dbl})
            n371 = Subtract(x=w66, y=w65) -> (x-y=w63:cluster{dbl, dbl})
            n372 = property on="disco1" class="Bool (strict)"("Position"=w63) -> ()  [unwired: 2 in, 2 out]
          }
        }
      }
      event Mouse Up {
        n373 = event-data() -> ()  [unwired: 1 in, 8 out]
        n374 = property on="Torre 2" class="Bool (strict)"() -> ("Bounds"=w105:T3)  [unwired: 2 in, 2 out]
        n375 = property on="Torre 2" class="Bool (strict)"() -> ("Position"=w104:T1)  [unwired: 2 in, 2 out]
        n376 = property on="disco1" class="Bool (strict)"() -> ("Position"=w78:T1)  [unwired: 2 in, 2 out]
        n377 = property on="disco1" class="Bool (strict)"() -> ("Bounds"=w77:T3)  [unwired: 2 in, 2 out]
        n378 = Add(x=w105, y=w104) -> (x+y=w103:T3)
        n379 = Add(x=w77, y=w78) -> (x+y=w108:T3)
        n380 = Less?(x=w104, y=w108) -> (x < y?=w107:cluster{bool, bool})
        n381 = Greater?(x=w103, y=w78) -> (0:w106:cluster{bool, bool})
        n382 = Unbundle(w107) -> (w112:bool, w111:bool)
        n383 = Unbundle(w106) -> (w114:bool, w113:bool)
        n384 = And(x=w112, y=w111) -> (x .and. y?=w109:bool)
        n385 = And(x=w114, y=w113) -> (x .and. y?=w110:bool)
        n386 = property on="Torre 3" class="Bool (strict)"() -> ("Position"=w91:T1)  [unwired: 2 in, 2 out]
        n387 = property on="Torre 3" class="Bool (strict)"() -> ("Bounds"=w92:T3)  [unwired: 2 in, 2 out]
        n388 = And(x=w109, y=w110) -> (x .and. y?=w70:bool)
        n389 = Not(x=w70) -> (.not. x?=w74:bool)
        n390 = Add(x=w92, y=w91) -> (x+y=w102:T3)
        n391 = Add(x=w77, y=w78) -> (x+y=w99:T3)
        n392 = Less?(x=w91, y=w99) -> (x < y?=w100:cluster{bool, bool})
        n393 = Greater?(x=w102, y=w78) -> (0:w101:cluster{bool, bool})
        n394 = Unbundle(w100) -> (w95:bool, w96:bool)
        n395 = Unbundle(w101) -> (w93:bool, w94:bool)
        n396 = property on="Torre 1" class="Bool (strict)"() -> ("Bounds"=w80:T3)  [unwired: 2 in, 2 out]
        n397 = property on="Torre 1" class="Bool (strict)"() -> ("Position"=w79:T1)  [unwired: 2 in, 2 out]
        n398 = And(x=w95, y=w96) -> (x .and. y?=w98:bool)
        n399 = And(x=w93, y=w94) -> (x .and. y?=w97:bool)
        n400 = And(x=w98, y=w97) -> (x .and. y?=w69:bool)
        n401 = Not(x=w69) -> (.not. x?=w75:bool)
        n402 = Add(x=w80, y=w79) -> (x+y=w81:T3)
        n403 = Add(x=w77, y=w78) -> (x+y=w84:T3)
        n404 = Less?(x=w79, y=w84) -> (x < y?=w83:cluster{bool, bool})
        n405 = Greater?(x=w81, y=w78) -> (0:w82:cluster{bool, bool})
        n406 = Unbundle(w83) -> (w88:bool, w87:bool)
        n407 = Unbundle(w82) -> (w90:bool, w89:bool)
        n408 = And(x=w88, y=w87) -> (x .and. y?=w85:bool)
        n409 = And(x=w90, y=w89) -> (x .and. y?=w86:bool)
        n410 = And(x=w85, y=w86) -> (x .and. y?=w68:bool)
        n411 = Not(x=w68) -> (.not. x?=w76:bool)
        n412 = Compound Arithmetic op=XOR(w74, w75, w76) -> (w73:bool)
        n413 = case shown="True" w73 {
          tunnel: [FALSE ("Accepted?") TRUE ("Accepted?")] -> w72
          frame False {
          }
          frame True {
            n414 = local read "Position 1"() -> (w117:T1)
            n415 = property on="disco1" class="Bool (strict)"("Position"=w117) -> ()  [unwired: 2 in, 2 out]
          }
        }
        n416 = Exclusive Or(1:w72, 2:w73) -> (0:w71:bool)
      }
      event Mouse Down {
        n417 = event-data() -> ("Coords"=w129:T2)  [unwired: 1 in, 7 out]
        n418 = property on="disco1" class="Bool (strict)"() -> ("Position"=w119:T1)  [unwired: 2 in, 2 out]
        "Position 1" <- w119
        n419 = property on="disco1" class="Bool (strict)"() -> ("Bounds"=w118:T3)  [unwired: 2 in, 2 out]
        n420 = Greater?(x=w129, y=w119) -> (0:w128:cluster{bool, bool})
        n421 = Unbundle(w128) -> (w124:bool, w123:bool)
        n422 = Add(x=w119, y=w118) -> (x+y=w130:T3)
        n423 = And(x=w124, y=w123) -> (x .and. y?=w121:bool)
        n424 = Less?(x=w129, y=w130) -> (x < y?=w127:cluster{bool, bool})
        n425 = Unbundle(w127) -> (w126:bool, w125:bool)
        n426 = And(x=w126, y=w125) -> (x .and. y?=w122:bool)
        n427 = And(x=w121, y=w122) -> (x .and. y?=w120:bool)
      }
    }
    n428 = property on="disco1" class="Bool (strict)"() -> ("Position"=→"Position":T1)  [unwired: 2 in, 2 out]
    n429 = case shown="True" "?" {
      frame False {
      }
      frame True {
        n430 = Equal?(x="seleccione  numero de discos", y=u16 3) -> (x = y?=w28:bool)
        "Boolean" <- w28
        n431 = Equal?(x="seleccione  numero de discos", y=u16 4) -> (x = y?=w26:bool)
        "Boolean 2" <- w26
        n432 = Equal?(x="seleccione  numero de discos", y=u16 5) -> (x = y?=w17:bool)
        "Boolean 3" <- w17
        n433 = Select(t=" disco 1 a torre 3\ndisco 2 a torre 2 \ndisco 1 a torre 2\ndisco 3 a torre 3\ndisco 1 a torre 1\ndisco 2 a torre 3\ndisco 1 a torre 3  ", s=w28, f="") -> (s? t:f=→"solucion del juego 3 discos":string)
        n434 = Select(t=" disco 1 a torre 2\ndisco 2 a torre 3\ndisco  1 a torre 3\ndisco 3 a torre 2\ndisco 1 a torre 1\ndisco 2 a torre 2\ndisco 1 a torre 2\ndisco 4 a torre 3\ndisco 1 a torre 3\ndisco 2 a torre 1 \ndisco 1 a torre 1\ndisco 3 a torre 3\ndisco 1 a torre 2\ndisco 2 a torre 3\ndisco 1 a torre 3", s=w26, f="") -> (s? t:f=→"Solucion del juego de 4 discos":string)
        n435 = Select(t="disco 1 a torre 3   -----  disco 1 a torre 2\ndisco 2 a torre 2    ----- disco 5 a torre 3\ndisco 1 a torre 2   ----- disco 1 a torre 1\ndisco 3 a torre 3   ----- disco 2 a torre 3\ndisco 1 a torre 1   -----  disco1 a torre 3\ndisco 2 a torre 3   -----  disco 3 a torre 2\n disco 1 a torre 3  ----- disco 1 a torre 2\ndisco 4 a torre 2   -----  disco 2 a torre 1\ndisco 1 a torre 2  ----- disco 1 a torre 1\ndisco 2 a torre 1  -----  disco 4 a torre 3\ndisco 1 a torre 1  -----  disco 1 a torre 3\ndisco 3 a torre 2  ----- disco 2 a torre 2\ndisco 1 a torre 3  -----  disco 1 a torre 2\ndisco 2 a torre 2  ----- disco 3 a torre 3\n                                       disco 1 a torre 1\n                                       disco 2 a torre 3 \n                                       disco 1 a torre 1", s=w17, f=" ") -> (s? t:f=→"Solucion del juego de 5 discos":string)
        n436 = case shown="5" "seleccione  numero de discos" {
          frame 0, Default {
          }
          frame 5 {
            n437 = property on="disco3" class="Bool (strict)"("Visible"=TRUE) -> ()  [unwired: 2 in, 2 out]
            n438 = property on="disco4" class="Bool (strict)"("Visible"=TRUE) -> ()  [unwired: 2 in, 2 out]
            n439 = property on="disco2" class="Bool (strict)"("Visible"=TRUE) -> ()  [unwired: 2 in, 2 out]
            n440 = property on="disco1" class="Bool (strict)"("Visible"=TRUE) -> ()  [unwired: 2 in, 2 out]
            n441 = property on="disco5" class="Bool (strict)"("Visible"=TRUE) -> ()  [unwired: 2 in, 2 out]
            n442 = property on="disco4" class="Bool (strict)"("Position"=T1 {"Left"=285, "Top"=429}) -> ()  [unwired: 2 in, 2 out]
            n443 = property on="disco5" class="Bool (strict)"("Position"=T1 {"Left"=271, "Top"=451}) -> ()  [unwired: 2 in, 2 out]
            n444 = property on="disco3" class="Bool (strict)"("Position"=T1 {"Left"=297, "Top"=405}) -> ()  [unwired: 2 in, 2 out]
            n445 = property on="disco2" class="Bool (strict)"("Position"=T1 {"Left"=309, "Top"=381}) -> ()  [unwired: 2 in, 2 out]
            n446 = property on="disco1" class="Bool (strict)"("Position"=T1 {"Left"=321, "Top"=356}) -> ()  [unwired: 2 in, 2 out]
          }
          frame 4 {
            n447 = property on="disco3" class="Bool (strict)"("Visible"=TRUE) -> ()  [unwired: 2 in, 2 out]
            n448 = property on="disco4" class="Bool (strict)"("Visible"=TRUE) -> ()  [unwired: 2 in, 2 out]
            n449 = property on="disco2" class="Bool (strict)"("Visible"=TRUE) -> ()  [unwired: 2 in, 2 out]
            n450 = property on="disco1" class="Bool (strict)"("Visible"=TRUE) -> ()  [unwired: 2 in, 2 out]
            n451 = property on="disco5" class="Bool (strict)"("Visible"=FALSE) -> ()  [unwired: 2 in, 2 out]
            n452 = property on="disco4" class="Bool (strict)"("Position"=T1 {"Left"=285, "Top"=441}) -> ()  [unwired: 2 in, 2 out]
            n453 = property on="disco5" class="Bool (strict)"("Position"=T1 {"Left"=69, "Top"=489}) -> ()  [unwired: 2 in, 2 out]
            n454 = property on="disco3" class="Bool (strict)"("Position"=T1 {"Left"=297, "Top"=417}) -> ()  [unwired: 2 in, 2 out]
            n455 = property on="disco2" class="Bool (strict)"("Position"=T1 {"Left"=309, "Top"=393}) -> ()  [unwired: 2 in, 2 out]
            n456 = property on="disco1" class="Bool (strict)"("Position"=T1 {"Left"=321, "Top"=368}) -> ()  [unwired: 2 in, 2 out]
          }
          frame 3 {
            n457 = property on="disco3" class="Bool (strict)"("Visible"=TRUE) -> ()  [unwired: 2 in, 2 out]
            n458 = property on="disco4" class="Bool (strict)"("Visible"=FALSE) -> ()  [unwired: 2 in, 2 out]
            n459 = property on="disco2" class="Bool (strict)"("Visible"=TRUE) -> ()  [unwired: 2 in, 2 out]
            n460 = property on="disco1" class="Bool (strict)"("Visible"=TRUE) -> ()  [unwired: 2 in, 2 out]
            n461 = property on="disco5" class="Bool (strict)"("Visible"=FALSE) -> ()  [unwired: 2 in, 2 out]
            n462 = property on="disco4" class="Bool (strict)"("Position"=T1 {"Left"=93, "Top"=477}) -> ()  [unwired: 2 in, 2 out]
            n463 = property on="disco5" class="Bool (strict)"("Position"=T1 {"Left"=81, "Top"=501}) -> ()  [unwired: 2 in, 2 out]
            n464 = property on="disco3" class="Bool (strict)"("Position"=T1 {"Left"=297, "Top"=441}) -> ()  [unwired: 2 in, 2 out]
            n465 = property on="disco2" class="Bool (strict)"("Position"=T1 {"Left"=309, "Top"=417}) -> ()  [unwired: 2 in, 2 out]
            n466 = property on="disco1" class="Bool (strict)"("Position"=T1 {"Left"=321, "Top"=392}) -> ()  [unwired: 2 in, 2 out]
          }
        }
      }
    }
  }
